vi "linux_command.vi"   [LabVIEW 2019]
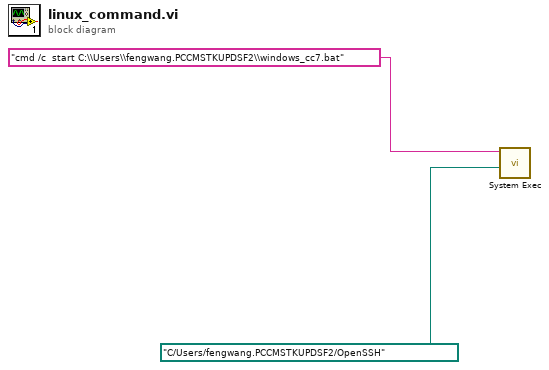
[diagram p0: block diagram]
diagram:
  n1 = call <vilib>:"System Exec.vi"("working directory"=path "C:/Users/fengwang.PCCMSTKUPDSF2/OpenSSH", "command line"="cmd /c  start C:\\Users\\fengwang.PCCMSTKUPDSF2\\windows_cc7.bat") -> ()  [unwired: 6 in, 4 out]
